vi "HexDAQ.vi"() -> ()   [LabVIEW 2016]
doc: "This is the main VI for the HexDAQ project. Contains the front panel controls steers the entire data taking, logging and display."
uses:
  input_params.ctl
  refs_front_panel.ctl
  <extravilib>/ChannelInstances/Tag-a[.](c(a[.](stamp),a[.](dbl)))/Read With Abort.vi
  <extravilib>/ChannelInstances/Tag-bool/Read With Abort.vi
  <extravilib>/ChannelInstances/Tag-t'input_params.ctl'/Write With Abort.vi
  <extravilib>/ChannelInstances/Tag-str/Write With Abort.vi
  <extravilib>/ChannelInstances/Tag-bool/Write With Abort.vi
  <extravilib>/ChannelInstances/Tag-t'data_env.ctl'/Instantiate.vi
  <extravilib>/ChannelInstances/Tag-t'input_params.ctl'/Instantiate.vi
  <extravilib>/ChannelInstances/Tag-str/Instantiate.vi
  <extravilib>/ChannelInstances/Tag-a[.](c(a[.](stamp),a[.](dbl)))/Instantiate.vi
  <extravilib>/ChannelInstances/Tag-bool/Instantiate.vi
  <extravilib>/ChannelInstances/Tag-a[.](c(a[.](stamp),a[.](dbl)))/EndpointRead.vi
  <extravilib>/ChannelInstances/Tag-bool/EndpointRead.vi
  <extravilib>/ChannelInstances/Tag-t'input_params.ctl'/Endpoint.vi
  <extravilib>/ChannelInstances/Tag-str/Endpoint.vi
  <extravilib>/ChannelInstances/Tag-bool/Endpoint.vi
  <extravilib>/ChannelInstances/Tag-bool.lvlib
  <extravilib>/ChannelInstances/Tag-a[.](c(a[.](stamp),a[.](dbl))).lvlib
  <extravilib>/ChannelInstances/Tag-str.lvlib
  user32.dll
  <extravilib>/ChannelInstances/Tag-t'input_params.ctl'.lvlib
panel:
  in  "Mask pad above (uA)":dbl=1.0
  in  "Mask pads":string
  in  "Source interlock?":bool=TRUE
  out "Missing current [%]\n(Sum cells - tot)/tot":dbl format="%#.0f"
  in  "Abort 3":bool
  in  "END DAQ 2":bool
  in  "Polarity: switch only affects contact test to be forward bias always.":enum32{"Radio Selection 1", "Radio Selection 2"}(radio)
  in  "CV Switch Delay (s)":dbl=0.3
  in  "IV Switch Delay (s)":dbl=0.3
  in  "CV voltage file":path=path "C:/Users/Administrator/Desktop/HGCAL_sensor_tests/config/voltagesCV.txt"
  in  "IV voltage file":path=path "C:/Users/Administrator/Desktop/HGCAL_sensor_tests/config/voltagesIV.txt"
  in  "Abort 2":bool
  in  "No CV corrections":bool=TRUE
  in  "Total curr/vlt \nevery x pads":i32=10
  in  "Disable Switchcard":bool
  in  "Comments (saved in data file)":string
  in  "Needle?":bool
  out "Total current":cluster{i32[], dbl[]}[](graph) caption="XY Graph"
  in  "CV voltage delay (s)":dbl=20.0
  in  "Sensor type":T1(ring)
  in  "Custom pad scan":string
  in  "Measurement type":T2(ring)=enum."Debug"
  in  "Hex pad numbers?":bool=TRUE
  in  "?":refnum<k7>(container)
  in  "Custom\nvoltages IV":string
  out "Single channel IV/CV curve":cluster{"X array":dbl[], "Y array":dbl[]}[](graph) caption="XY Graph"
  in  "Repeat":i32=1
  in  "LCR signal voltage (V)":dbl=0.501
  in  "LCR signal frequenzy (kHz)":dbl=50.0 format="%#_13g"
  in  "Sampling number":i32=3
  in  "DMM device":T3(ring)=enum."Keithley6487"
  in  "Take environmental sensor data from":T4(ring)=enum."Switch Matrix"
  out "Environmental data":cluster{timestamp[], dbl[]}[](graph)
  out "Elapsed time":dbl format="%<%H:%M:%S>t"
  out "Estimated remaining time":dbl format="%<%H:%M:%S>t"
  out "Channel values":cluster{i32[], dbl[]}[](graph) caption="XY Graph"
  out "Current channel":dbl format="%#_13g"
  out "Current source voltage (V)":dbl format="%#_13g"
  in  "Abort":bool
  in  "Output file":refnum<k7>(container) caption="Preview data file"
  in  "END DAQ":bool
  in  "START DAQ":bool
  in  "Custom\nvoltages CV":string
  in  "Data storage location:":path=path "C:/Users/Administrator/cernbox/HGCAL test results/Data"
  in  "Plot after execution?":bool=TRUE
  in  "Voltage limit (V)":dbl=1000.0
  in  "Compliance  level (uA)":dbl=500.0
  in  "VISA resource name LCR":refnum<visa-resource-name>="LCR_E4980"
  in  "VISA resource name DMM":refnum<visa-resource-name>="KEITHLEY_6487"
  in  "VISA resource name source":refnum<visa-resource-name>="Source_2410"
  in  "IV voltage delay (s)":dbl=5.0
  in  "Display/needle\nchannel":i32=144
  in  "Open after execution?":bool
  in  "Identifier (eg. wafer number)":string="Debug"
  # "HexDAQ\nThe LabVIEW program for HGCAL sensor tests\nFeedback and bug reports to andreas.alexander.maier@cern.ch"
  # "Measurement settings"
  # "Bookkeeping settings"
  # "VISA settings"
  # "Both used to determine \nthe folder and file names"
  # "Device settings"
  # "Debug settings"
  # "Timing settings"
  # "Data processing settings"
  # "Ctrl+H for full display"
  # "p on n (no sign inversion)"
  # "n on p (inversion for contact test)"
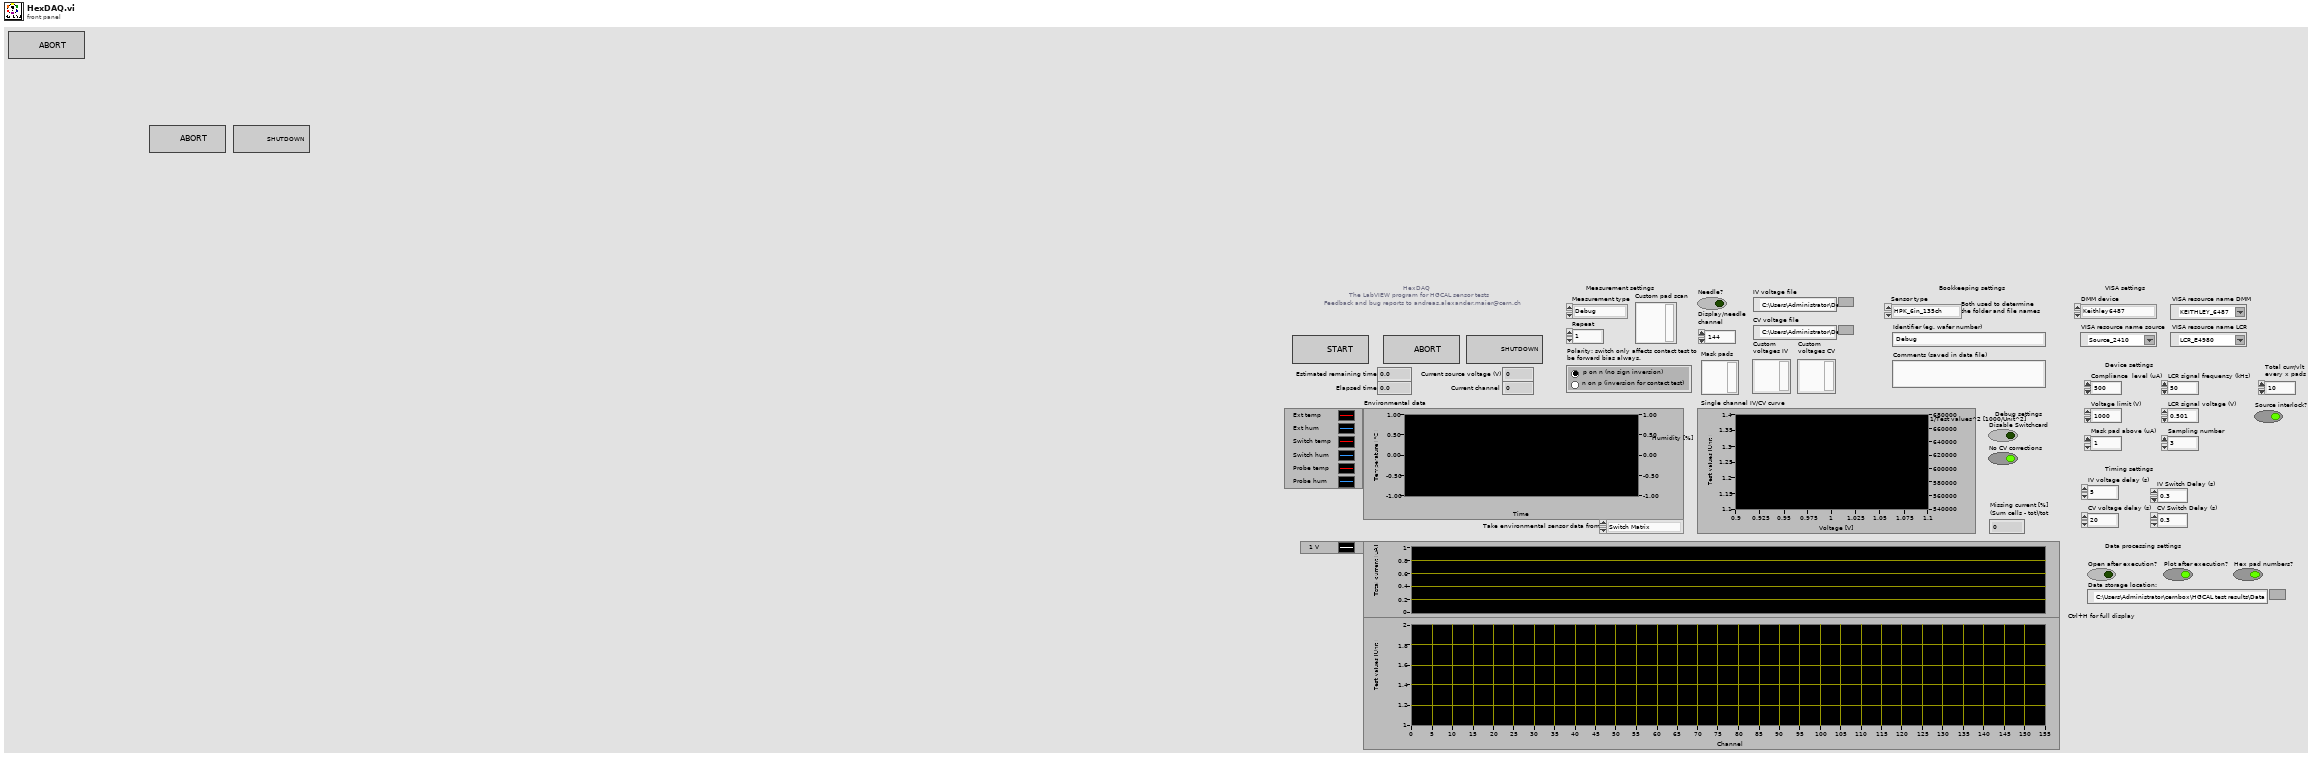
[diagram p1: front panel]
types:
  T1 = enum16{"HPK_6in_135ch", "HPK_8in_271ch", "IFX_8in_256ch", "Diode", "HPK_6in_239ch", "Full_Matrix"}
  T2 = enum16{"IV", "CV", "Debug", "Test_contact", "IV+CV"}
  T3 = enum16{"Keithley2001", "Keithley2450", "Keithley2410", "Keithley6487", "Keithley6517"}
  T4 = enum16{"Sensirion sht1x/7x", "Switch Matrix", "Probecard"}
  T5 = typedef "refs_front_panel.ctl" = cluster{"Current voltage (V)":refnum<vi>, "Elapsed time":refnum<vi>, "Current channel":refnum<vi>, "Abort":refnum<vi>, "Estimated remaining time":refnum<vi>, "Channel values XYGraph":refnum<vi>, "Single channel XYGraph":refnum<vi>, "Total current XYGraph":refnum<vi>, "Missing\ncurrent [%]":refnum<vi>}
  T6 = typedef "input_params.ctl" = cluster{"Measurement type":enum16{"IV", "CV", "Debug", "Test_contact"}, "Sensor type":enum16{"HPK_6in_135ch", "HPK_8in_271ch", "IFX_8in_256ch", "Diode", "HPK_6in_239ch", "Full_Matrix", ""}, "Identifier":string, "Open after execution?":bool, "Plot after execution?":bool, "Display channel":i32, "Voltage Delay (s)":dbl, "Switch Delay (s)":dbl, "VISA resource name source":refnum<visa-resource-name>, "VISA resource name DMM":refnum<visa-resource-name>, "VISA resource name LCR":refnum<visa-resource-name>, "Compliance  Level (A)":dbl, "Voltage Limit (V)":dbl, "Data storage location":string, "Scan voltages":string, "Use source as DMM?":bool, "LCR signal frequenzy (Hz)":dbl, "DMM device":enum16{"Keithley2001", "Keithley2450", "Keithley2410", "Keithley6487", "Keithley6517"}, "Sampling number":i32, "Use env. sensors on":enum16{"Sensirion sht1x/7x", "Switch Matrix", "Probecard"}, "Switchboard Handle":u32, "Use Switchboard":bool, "LCR signal voltage (V)":dbl, "Repeat":i32, "Scan voltages IV":string, "Scan voltages CV":string, "Hex pad numbers?":bool, "Set measurement type":enum16{"IV", "CV", "Debug", "Test_contact", "IV+CV"}, "Custom pad scan":string, "IV voltage Delay (s)":dbl, "CV voltage Delay (s)":dbl, "Needle measurement?":bool, "Comments":string, "LCR signal frequenzy (kHz)":dbl, "Compliance  Level (uA)":dbl, "Open Correction Array":dbl[][], "Current set voltage":dbl, "Last set voltage":dbl, "Current channel":i32, "Last OpenCorrection index":i32, "Total curr/vltg every x steps":i32, "Current channel iteration":i32, "No CV corrections":bool, "Mapfile":string, "Corrfile":string, "IV voltage file":path, "CV voltage file":path, "IV Switch Delay (s)":dbl, "CV Switch Delay (s)":dbl, "Invert polarity":bool, "Set debug dirs":bool, "Is n on p":bool, "Source interlock?":bool, "Voltage file used?":bool, "Pad mask":string, "Mask pad above (uA)":dbl}
  T7 = typedef "Tag-t'input_params.ctl'.lvlib/))Channel.ctl" = refnum<queue>
  T8 = typedef "Tag-str.lvlib/))Channel.ctl" = refnum<queue>
  T9 = typedef "data_dynamic.ctl" = cluster{"Output file":path, "Y-label text":string, "Current set voltage":dbl, "Set voltage column":dbl[], "Pad number column":dbl[], "Data  column":dbl[], "Number of voltages":i32, "Compliance current (A)":dbl, "Geofile":string, "Peak voltage":dbl, "Hex PDF file":string, "Voltage array":dbl[], "Total current column":dbl[], "Timestamp column":dbl[], "Data name":string, "Data unit":string, "2nd data column":dbl[], "2nd data name":string, "2nd data unit":string, "3rd data column":dbl[], "4th data column":dbl[], "3rd data name":string, "3rd data unit":string, "4th data name":string, "4th data unit":string, "Actual voltage column":dbl[], "2nd Y-label text":string, "Single channel plot":path, "Temperature column":dbl[], "Humidity column":dbl[], "Channel switch array":i32[], "1st single plot name":string, "2nd single plot name":string, "All channels plot":path, "HexPlot command":string, "Custom channel array":i32[], "Data  error column":dbl[], "2nd data  error column":dbl[], "3rd data error column":dbl[], "4th data  error column":dbl[], "Total current plot":path, "5th data column":dbl[], "5th data  error column":dbl[], "6th data column":dbl[], "6th data  error column":dbl[], "5th data name":string, "5th data unit":string, "6th data name":string, "6th data unit":string, "HexPlot matrix command":string}
  T10 = typedef "Tag-bool.lvlib/))Channel.ctl" = refnum<queue>
  T11 = typedef "Tag-a[.](c(a[.](stamp),a[.](dbl))).lvlib/))Channel.ctl" = refnum<queue>
  T12 = typedef "Tag-t'data_env.ctl'.lvlib/))Channel.ctl" = refnum<queue>
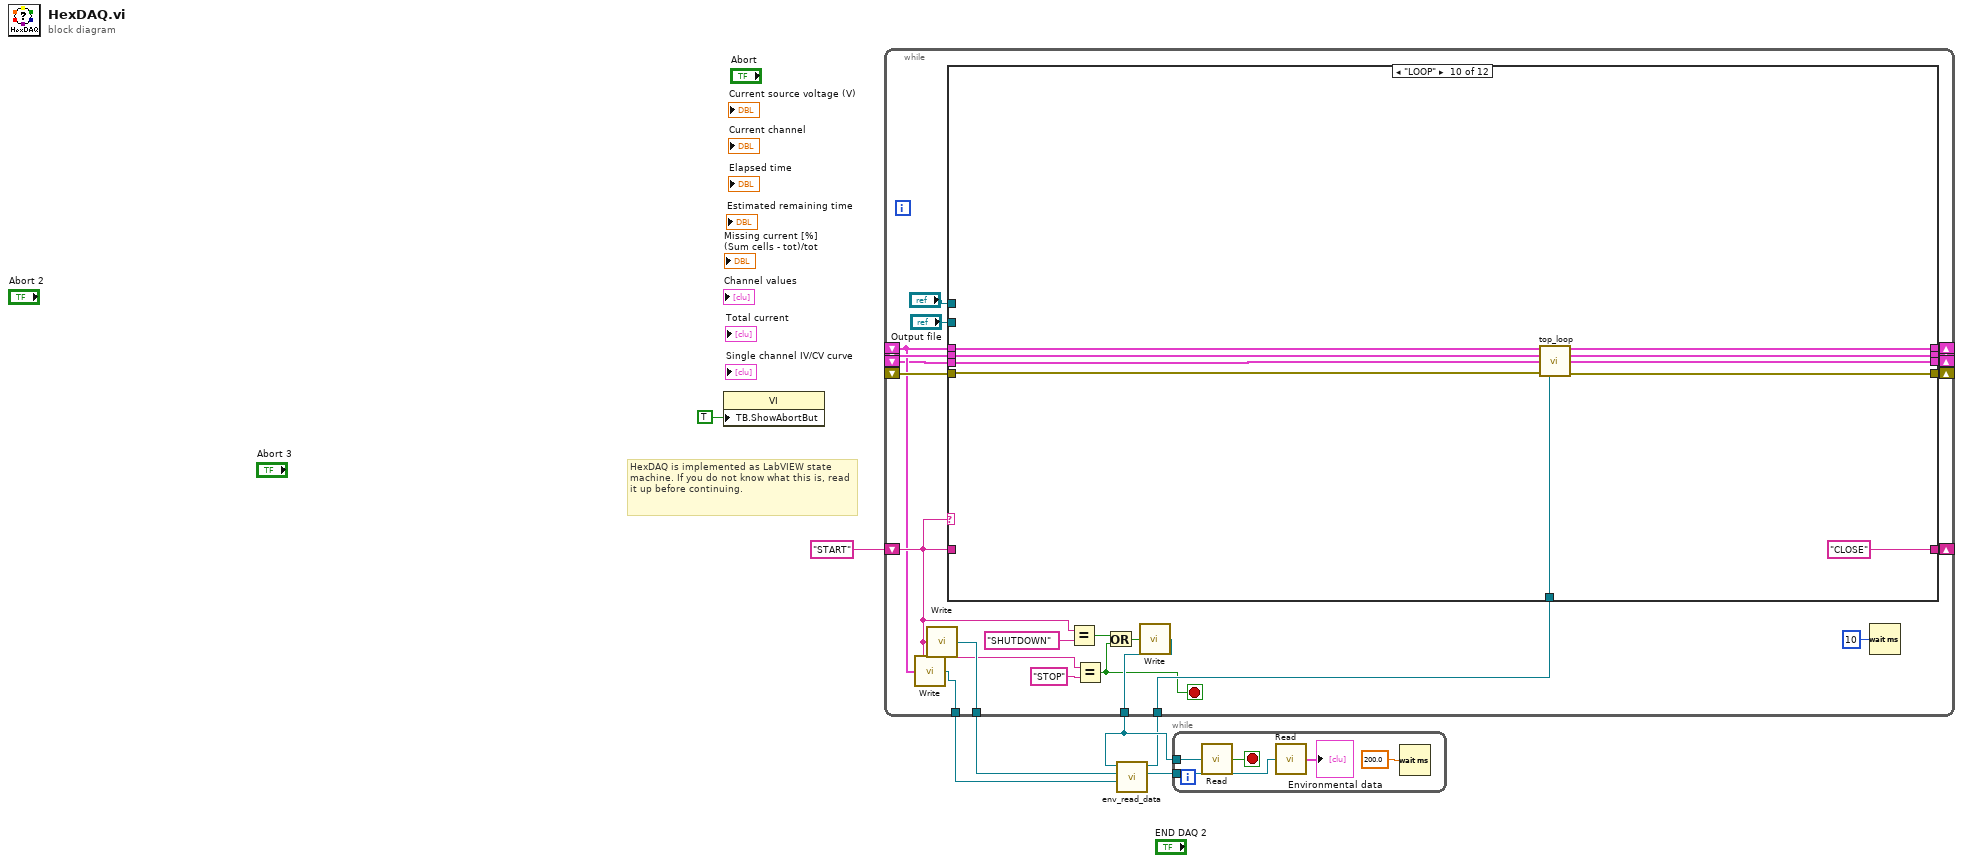
[diagram p0: block diagram]
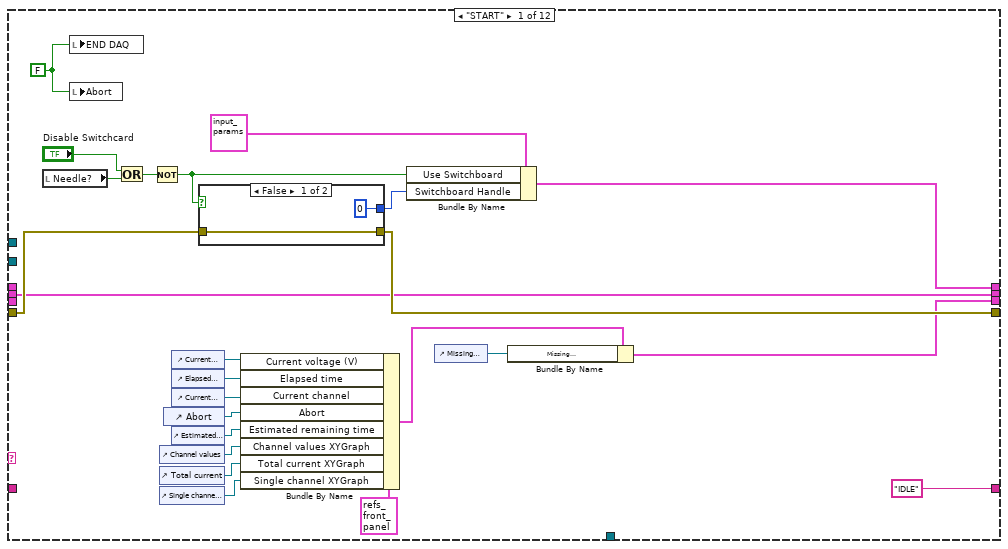
[diagram p2: hidden frame]
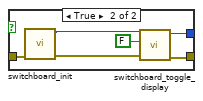
[diagram p3: hidden frame]
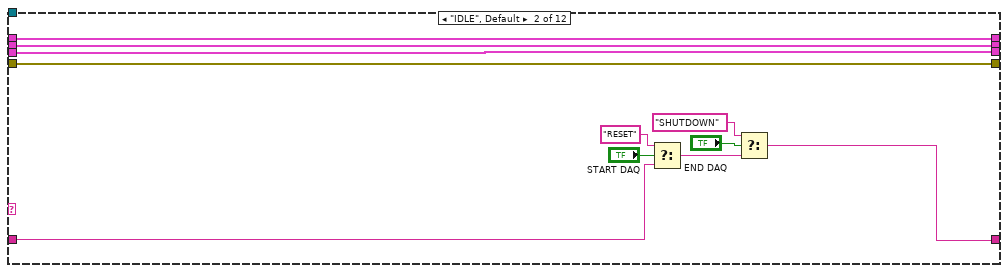
[diagram p4: hidden frame]
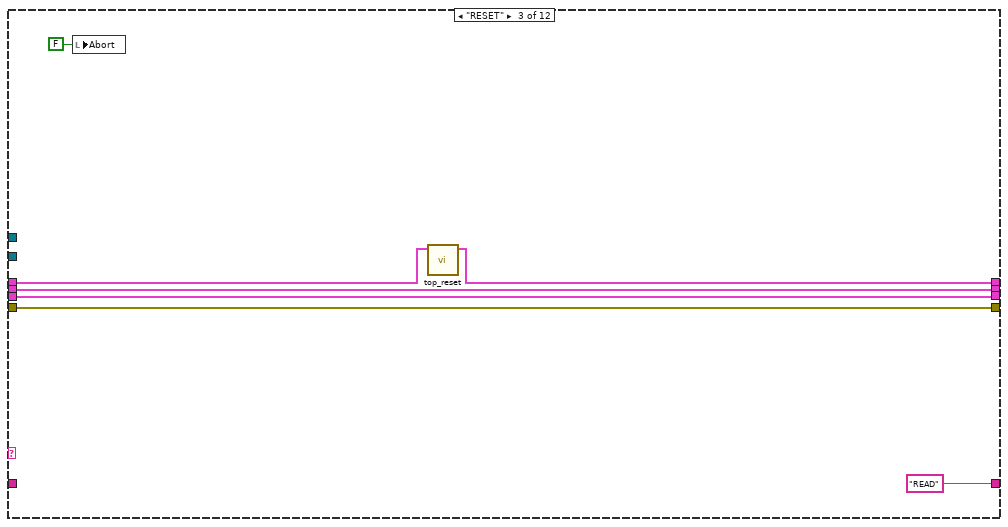
[diagram p5: hidden frame]
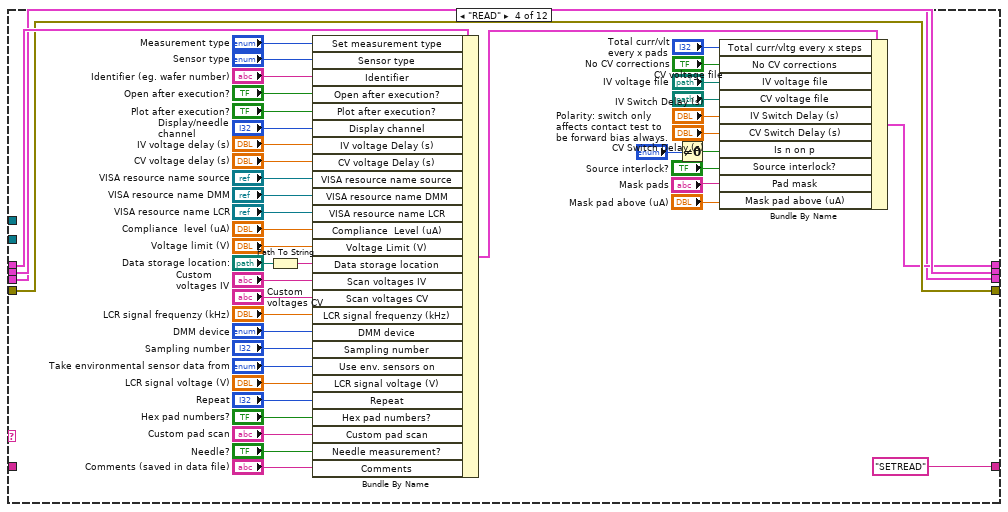
[diagram p6: hidden frame]
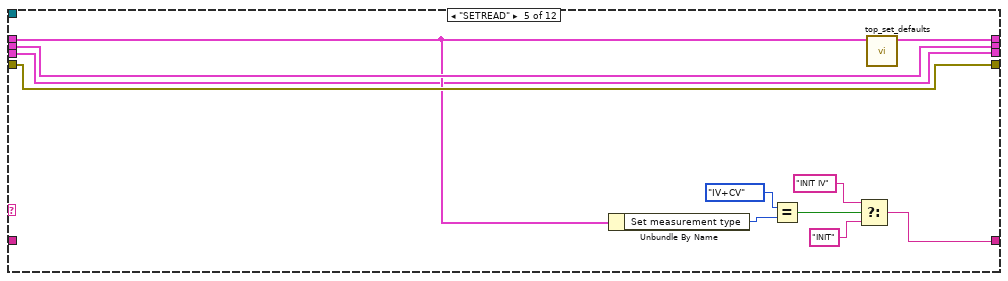
[diagram p7: hidden frame]
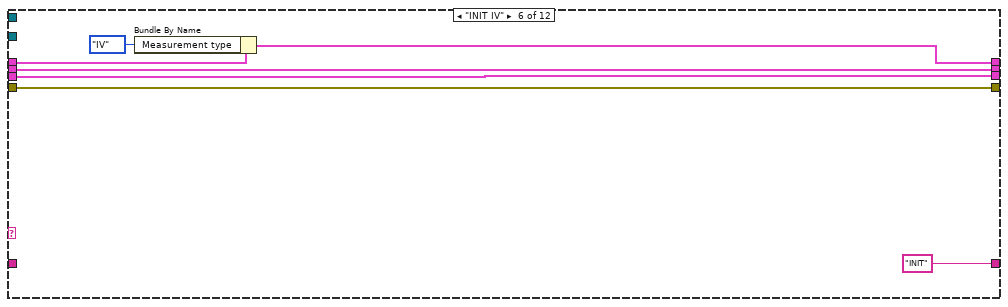
[diagram p8: hidden frame]
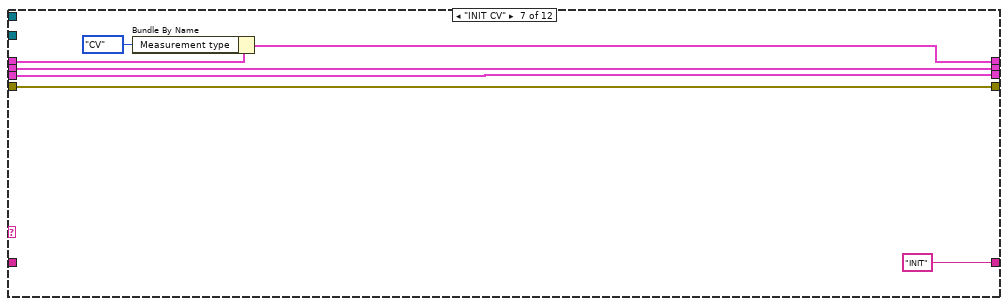
[diagram p9: hidden frame]
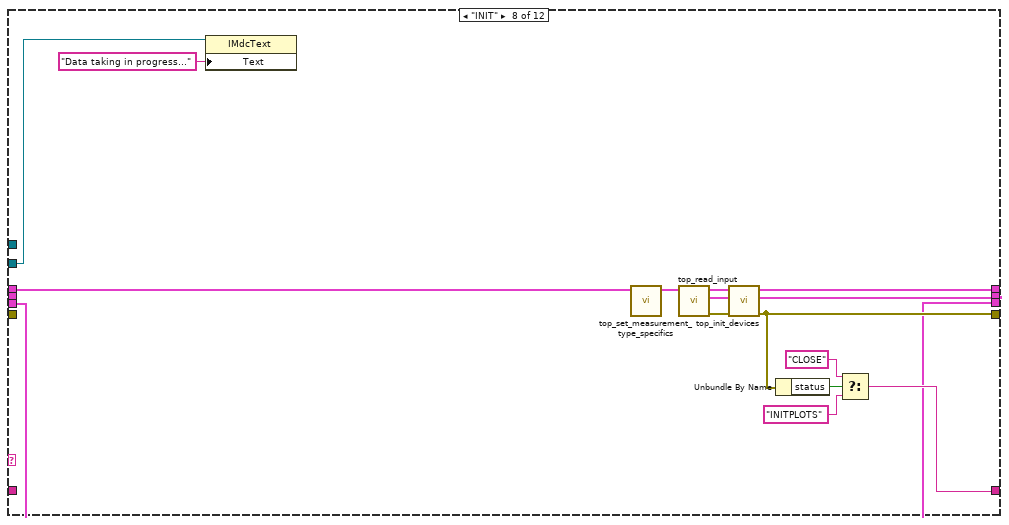
[diagram p10: hidden frame]
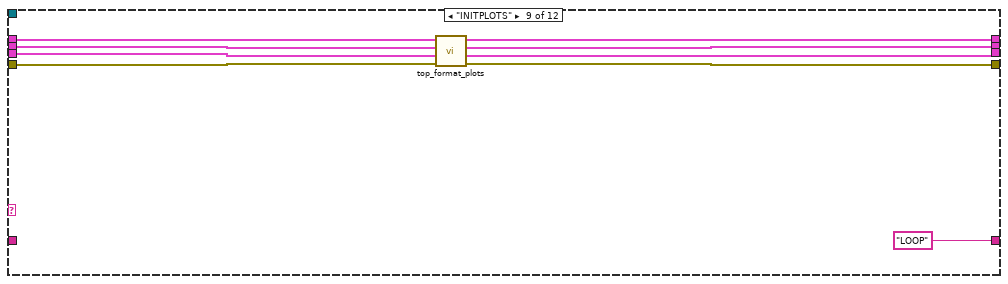
[diagram p11: hidden frame]
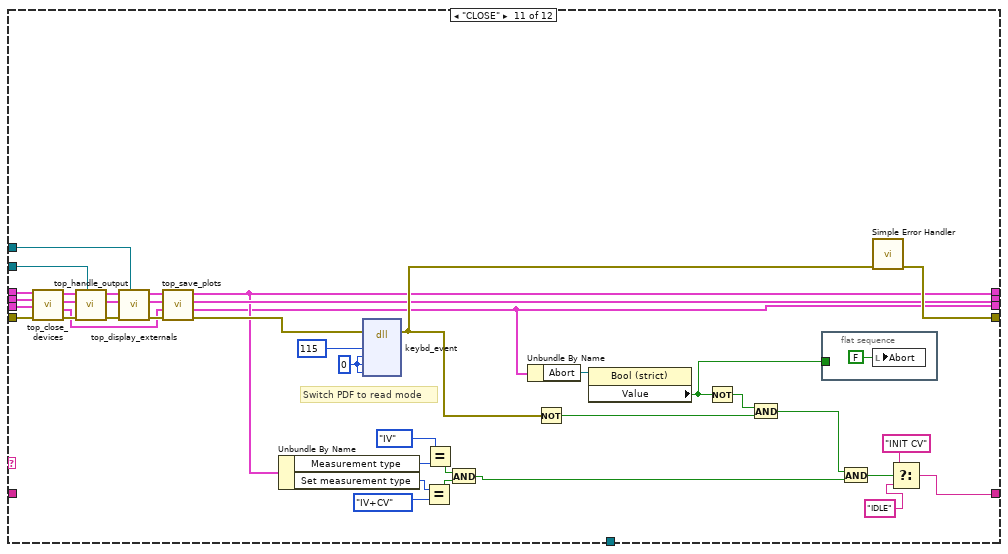
[diagram p12: hidden frame]
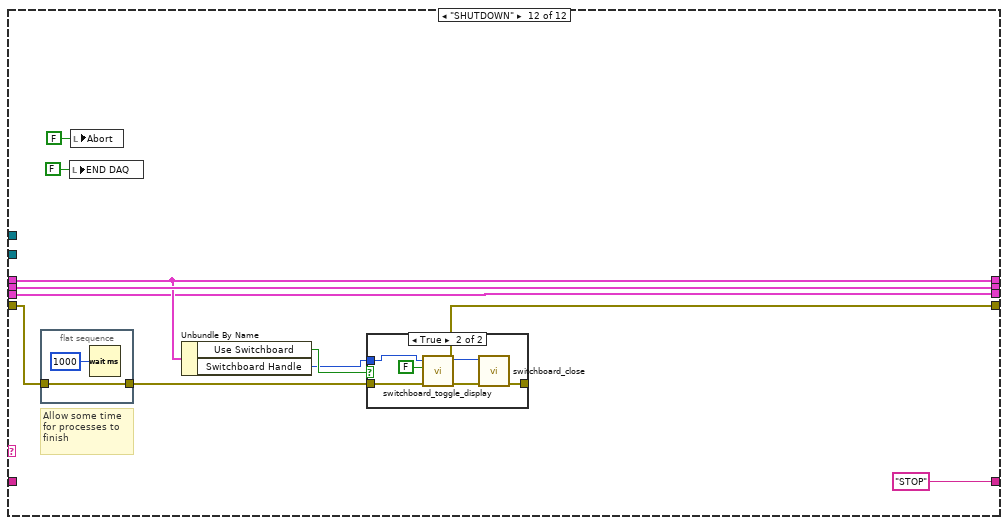
[diagram p13: hidden frame]
diagram:
  # "HexDAQ is implemented as LabVIEW state machine. If you do not know what this is, read it up before continuing."
  n1 = property class="VI"("TB.ShowAbortBut"=TRUE ("Tool Bar:Show Abort Button")) -> ()  [unwired: 2 in, 2 out]
  n2 = while {
    shift-right: [w29] -> _
    shift-left: "START" -> [w16]
    shift-right: [w24] -> _
    shift-left: _ -> [w22]
    shift-right: [w26] -> _
    shift-left: _ -> [w23]
    shift-right: [w25] -> _
    shift-left: _ -> [w12]
    tunnel: [w21] -> w5
    tunnel: w1 -> [w19]
    tunnel: [w18] -> w3
    tunnel: [w8] -> w2
    shift-right: [w10] -> _
    shift-left: _ -> [w9]
    stop <- w13 stop-if-true
    n3 = call <extravilib>:"Write.vi"("element"=w12) -> ("channel"=w8:T7)  [unwired: 1 out]
    n4 = call <extravilib>:"Write.vi"("element"=w16) -> ("channel"=w18:T8)  [unwired: 1 out]
    n5 = case shown="\"LOOP\"" w16 {
      tunnel: w16 -> [_ w72 _ _ _ _ _ _ _ _ _ _]
      tunnel: ["IDLE" ("t") w69 "READ" ("t") "SETREAD" ("t") w130 "INIT" ("t") "INIT" ("t") w153 "LOOP" ("t") "CLOSE" ("t") w202 "STOP" ("t")] -> w29
      tunnel: [w47 w65 w74 w92 w127 w139 w146 w161 w169 w182 w192 w227] -> w25
      tunnel: [w51 w64 w78 w102 w134 w142 w149 w157 w165 w180 w215 w231] -> w24
      tunnel: [w48 w63 w75 w103 w135 w141 w148 w160 w168 w181 w194 w234] -> w26
      tunnel: w12 -> [_ w65 w73 w104 w126 w140 w147 w151 w172 w177 w217 w227]
      tunnel: w23 -> [w48 w63 w75 w103 w135 w141 w148 _ w173 w178 w212 w234]
      tunnel: w22 -> [w52 w64 w78 w102 w134 w142 w149 _ w166 w179 w216 w229]
      tunnel: "Output file" -> [_ _ _ _ _ _ _ w158 _ _ w214 _]
      tunnel: "?" -> [_ _ _ _ _ _ _ _ _ _ w213 _]
      tunnel: w19 -> [_ _ _ _ _ _ _ _ _ w176 _ _]
      tunnel: [w32 w62 w77 w89 w125 w136 w143 w152 w167 w175 w191 w226] -> w10
      tunnel: w9 -> [_ w62 w77 w89 w125 w136 w143 w152 w170 w174 w185 w226]
      frame "START" {
        w33 = FALSE ("Abort")
        n6 = local read "Needle?"() -> (w44:bool)
        n7 = local write "END DAQ"(w33) -> ()
        n8 = local write "Abort"(w33) -> ()
        n9 = Or(x="Disable Switchcard", y=w44) -> (x .or. y?=w43:bool)
        n10 = Not(x=w43) -> (.not. x?=w46:bool)
        n11 = control-ref of="Channel values"() -> (w36:refnum<vi>)
        n12 = control-ref of="Total current"() -> (w35:refnum<vi>)
        n13 = control-ref of="Single channel IV/CV curve"() -> (w34:refnum<vi>)
        n14 = control-ref of="Abort"() -> (w38:refnum<vi>)
        n15 = control-ref of="Current source voltage (V)"() -> (w40:refnum<vi>)
        n16 = control-ref of="Elapsed time"() -> (w41:refnum<vi>)
        n17 = control-ref of="Current channel"() -> (w39:refnum<vi>)
        n18 = control-ref of="Estimated remaining time"() -> (w37:refnum<vi>)
        n19 = case shown="False" w46 {
          tunnel: w52 -> [w55 w61]
          tunnel: [w55 w60] -> w51
          tunnel: [u32 0 ("Handle") w58] -> w50
          frame False {
          }
          frame True {
            n20 = call <instrlib>:"switchboard_init.vi"("error in"=w61) -> ("error out"=w57:errorcluster, "Handle"=w56:u32)  [unwired: 9 in]
            n21 = call <instrlib>:"switchboard_toggle_display.vi"("error in"=w57, "On/Off"=FALSE, "Handle"=w56) -> ("error out"=w60:errorcluster, "Handle out"=w58:u32)  [unwired: 7 in]
          }
        }
        n22 = Bundle By Name(cluster=T5 {"Current voltage (V)"=refnum, "Elapsed time"=refnum, "Current channel"=refnum, "Abort"=refnum, "Estimated remaining time"=refnum, "Channel values XYGraph"=refnum, "Single channel XYGraph"=refnum, "Total current XYGraph"=refnum, "Missing\ncurrent [%]"=refnum} ("Cluster"), "Current voltage (V)"=w40, "Elapsed time"=w41, "Current channel"=w39, "Abort"=w38, "Estimated remaining time"=w37, "Channel values XYGraph"=w36, "Total current XYGraph"=w35, "Single channel XYGraph"=w34) -> (w31:T5)
        n23 = Bundle By Name(cluster=T6 {"Measurement type"=enum."Debug", "Sensor type"=enum."HPK_6in_135ch", "Identifier"="test.txt", "Open after execution?"=FALSE, "Plot after execution?"=FALSE, "Display channel"=0, "Voltage Delay (s)"=0.5, "Switch Delay (s)"=0.01, "VISA resource name source"="", "VISA resource name DMM"="", "VISA resource name LCR"="", "Compliance  Level (A)"=10.0, "Voltage Limit (V)"=1000.0, "Data storage location"="", "Scan voltages"="", "Use source as DMM?"=FALSE, "LCR signal frequenzy (Hz)"=10.0, "DMM device"=enum."Keithley2001", "Sampling number"=1, "Use env. sensors on"=enum."Sensirion sht1x/7x", "Switchboard Handle"=0, "Use Switchboard"=FALSE, "LCR signal voltage (V)"=10000.0, "Repeat"=1, "Scan voltages IV"="", "Scan voltages CV"="", "Hex pad numbers?"=FALSE, "Set measurement type"=enum."Debug", "Custom pad scan"="", "IV voltage Delay (s)"=0.5, "CV voltage Delay (s)"=0.5, "Needle measurement?"=FALSE, "Comments"="test.txt", "LCR signal frequenzy (kHz)"=10.0, "Compliance  Level (uA)"=10.0, "Open Correction Array"=array2304x3[6912 elements], "Current set voltage"=0.0, "Last set voltage"=0.0, "Current channel"=0, "Last OpenCorrection index"=-1, "Total curr/vltg every x steps"=10, "Current channel iteration"=0, "No CV corrections"=FALSE, "Mapfile"="", "Corrfile"="", "IV voltage file"=path "", "CV voltage file"=path "", "IV Switch Delay (s)"=0.01, "CV Switch Delay (s)"=0.01, "Invert polarity"=FALSE, "Set debug dirs"=FALSE, "Is n on p"=FALSE, "Source interlock?"=TRUE, "Voltage file used?"=FALSE, "Pad mask"="", "Mask pad above (uA)"=1.0} ("Input parameters"), "Use Switchboard"=w46, "Switchboard Handle"=w50) -> (w47:T6)
        n24 = control-ref of="Missing current [%]\n(Sum cells - tot)/tot"() -> (w30:refnum<vi>)
        n25 = Bundle By Name(cluster=w31, "Missing\ncurrent [%]"=w30) -> (w32:T5)
      }
      frame "IDLE", Default {
        n26 = Select(t="RESET", s="START DAQ", f=w72) -> (s? t:f=w70:string)
        n27 = Select(t="SHUTDOWN", s="END DAQ", f=w70) -> (s? t:f=w69:string)
      }
      frame "RESET" {
        n28 = local write "Abort"(FALSE ("Abort")) -> ()
        n29 = call "top_reset.vi"("Input parameters"=w73) -> ("New input parameters"=w74:T6)  [unwired: 10 in]
      }
      frame "READ" {
        n30 = Path To String(path="Data storage location:") -> (string=w107:string)
        n31 = Bundle By Name(cluster=w104, "Set measurement type"="Measurement type", "Sensor type"="Sensor type", "Identifier"="Identifier (eg. wafer number)", "Open after execution?"="Open after execution?", "Plot after execution?"="Plot after execution?", "Display channel"="Display/needle\nchannel", "IV voltage Delay (s)"="IV voltage delay (s)", "CV voltage Delay (s)"="CV voltage delay (s)", "VISA resource name source"="VISA resource name source", "VISA resource name DMM"="VISA resource name DMM", "VISA resource name LCR"="VISA resource name LCR", "Compliance  Level (uA)"="Compliance  level (uA)", "Voltage Limit (V)"="Voltage limit (V)", "Data storage location"=w107, "Scan voltages IV"="Custom\nvoltages IV", "Scan voltages CV"="Custom\nvoltages CV", "LCR signal frequenzy (kHz)"="LCR signal frequenzy (kHz)", "DMM device"="DMM device", "Sampling number"="Sampling number", "Use env. sensors on"="Take environmental sensor data from", "LCR signal voltage (V)"="LCR signal voltage (V)", "Repeat"="Repeat", "Hex pad numbers?"="Hex pad numbers?", "Custom pad scan"="Custom pad scan", "Needle measurement?"="Needle?", "Comments"="Comments (saved in data file)") -> (w93:T6)
        n32 = Not Equal To 0?(x="Polarity: switch only affects contact test to be forward bias always.") -> (x != 0?=w84:bool)
        n33 = Bundle By Name(cluster=w93, "Total curr/vltg every x steps"="Total curr/vlt \nevery x pads", "No CV corrections"="No CV corrections", "IV voltage file"="IV voltage file", "CV voltage file"="CV voltage file", "IV Switch Delay (s)"="IV Switch Delay (s)", "CV Switch Delay (s)"="CV Switch Delay (s)", "Is n on p"=w84, "Source interlock?"="Source interlock?", "Pad mask"="Mask pads", "Mask pad above (uA)"="Mask pad above (uA)") -> (w92:T6)
      }
      frame "SETREAD" {
        n34 = Unbundle By Name(w126) -> ("Set measurement type"=w128:T2)
        n35 = Equal?(x=T2."IV+CV" ("Measurement type"), y=w128) -> (x = y?=w129:bool)
        n36 = Select(t="INIT IV", s=w129, f="INIT" ("t")) -> (s? t:f=w130:string)
        n37 = call "top_set_defaults.vi"("Input parameters"=w126) -> ("Input parameters out"=w127:T6)  [unwired: 10 in]
      }
      frame "INIT IV" {
        n38 = Bundle By Name(cluster=w140, "Measurement type"=enum16{"IV", "CV", "Debug", "Test_contact"}."IV") -> (w139:T6)
      }
      frame "INIT CV" {
        n39 = Bundle By Name(cluster=w147, "Measurement type"=enum16{"IV", "CV", "Debug", "Test_contact"}."CV") -> (w146:T6)
      }
      frame "INIT" {
        n40 = property class="IMdcText"(reference=w158, "Text"="Data taking in progress...") -> ()  [unwired: 1 in, 2 out]
        n41 = call "top_set_measurement_type_specifics.vi"("Input parameters"=w151) -> ("Input parameters out"=w150:T6)  [unwired: 10 in]
        n42 = call "top_read_input.vi"("Input parameters"=w150) -> ("error out"=w163:errorcluster, "Dynamic data"=w162:T9, "Input parameters"=w164:T6)  [unwired: 8 in]
        n43 = call "top_init_devices.vi"("error in (no error)"=w163, "Dynamic data"=w162, "Input parameters"=w164) -> ("error out"=w157:errorcluster, "Dynamic data"=w160:T9, "Input parameters"=w161:T6)  [unwired: 6 in]
        n44 = Unbundle By Name(w157) -> ("status"=w156:bool)
        n45 = Select(t="CLOSE", s=w156, f="INITPLOTS" ("t")) -> (s? t:f=w153:string)
      }
      frame "INITPLOTS" {
        n46 = call "top_format_plots.vi"("error in"=w166, "Front panel refs"=w170, "Dynamic data"=w173, "Input parameters"=w172) -> ("error out"=w165:errorcluster, "Front panel refs out"=w167:T5, "Dynamic data out"=w168:T9, "Input parameters out"=w169:T6)  [unwired: 4 in]
      }
      frame "LOOP" {
        n47 = call "top_loop.vi"("Input parameters"=w177, "Dynamic data"=w178, "Front_panel_refs"=w174, "error in (no error)"=w179, "Environmental data"=w176) -> ("Input parameters out"=w182:T6, "Dynamic data out"=w181:T9, "Front_panel_refs out"=w175:T5, "error out"=w180:errorcluster)  [unwired: 7 in]
      }
      frame "CLOSE" {
        w199 = u8 0 ("bScan")
        # "Switch PDF to read mode"
        n48 = call "top_close_devices.vi"("error in (no error)"=w216, "Front_panel_refs"=w185, "Dynamic data"=w212, "Input parameters"=w217) -> ("error out"=w223:errorcluster, "Front_panel_refs out"=w184:T5, "Dynamic data"=w221:T9, "Input parameters"=w222:T6)  [unwired: 4 in]
        n49 = call "top_handle_output.vi"("Output file text box"=w214, "error in (no error)"=w223, "Dynamic data"=w221, "Input parameters"=w222) -> ("error out"=w220:errorcluster, "Dynamic data"=w219:T9, "Input parameters"=w218:T6)  [unwired: 5 in]
        n50 = call "top_display_externals.vi"("AcroPDF"=w213, "error in (no error)"=w220, "Dynamic data"=w219, "Input parameters"=w218) -> ("error out"=w211:errorcluster, "Dynamic data"=w195:T9, "Input parameters"=w193:T6)  [unwired: 5 in]
        n51 = call "top_save_plots.vi"("error in"=w211, "Front_panel_refs"=w184, "Dynamic data"=w195, "Input parameters"=w193) -> ("error out"=w197:errorcluster, "Front_panel_refs out"=w191:T5, "Dynamic data out"=w194:T9, "Input parameters out"=w192:T6)  [unwired: 4 in]
        n52 = Unbundle By Name(w192) -> ("Measurement type"=w210:enum16{"IV", "CV", "Debug", "Test_contact"}, "Set measurement type"=w208:T2)
        n53 = dll-call lib="user32.dll" fn="keybd_event"(error in=w197, "bVk"=u8 115 ("Virtual Key"), "bScan"=w199, "dwFlags"=w199, "dwExtraInfo"=w199) -> (error out=w196:errorcluster)  [unwired: 7 in, 1 out]
        n54 = Equal?(x=w208, y=T2."IV+CV") -> (x = y?=w205:bool)
        n55 = Equal?(x=enum16{"IV", "CV", "Debug", "Test_contact"}."IV", y=w210) -> (x = y?=w206:bool)
        n56 = And(x=w206, y=w205) -> (x .and. y?=w187:bool)
        n57 = Unbundle By Name(w191) -> ("Abort"=w190:refnum<vi>)
        n58 = Not(x=w196) -> (.not. x?=w188:bool)
        n59 = property class="Bool (strict)"(reference=w190) -> ("Value"=w201:bool)  [unwired: 1 in, 2 out]
        n60 = Not(x=w201) -> (.not. x?=w189:bool)
        n61 = And(x=w189, y=w188) -> (x .and. y?=w186:bool)
        n62 = flat-sequence {
          tunnel: w201 -> [_]
          frame #0 {
            n63 = local write "Abort"(FALSE ("Abort")) -> ()
          }
        }
        n64 = And(x=w186, y=w187) -> (x .and. y?=w200:bool)
        n65 = call <vilib>:"Simple Error Handler.vi"("error in (no error)"=w196) -> ("error out"=w215:errorcluster)  [unwired: 4 in, 4 out]
        n66 = Select(t="INIT CV", s=w200, f="IDLE" ("t")) -> (s? t:f=w202:string)
      }
      frame "SHUTDOWN" {
        # "Allow some time\nfor processes to\nfinish"
        n67 = flat-sequence {
          tunnel: w229 -> [w236]
          tunnel: [w236] -> w228
          frame #0 {
            n68 = Wait (ms)(milliseconds to wait=u32 1000) -> ()  [unwired: 1 out]
          }
        }
        n69 = local write "END DAQ"(FALSE ("END DAQ")) -> ()
        n70 = local write "Abort"(FALSE ("Abort")) -> ()
        n71 = Unbundle By Name(w227) -> ("Use Switchboard"=w233:bool, "Switchboard Handle"=w232:u32)
        n72 = case shown="True" w233 {
          tunnel: w228 -> [w238 w242]
          tunnel: [w238 w244] -> w231
          tunnel: w232 -> [_ w241]
          frame False {
          }
          frame True {
            n73 = call <instrlib>:"switchboard_toggle_display.vi"("error in"=w242, "On/Off"=FALSE, "Handle"=w241) -> ("error out"=w239:errorcluster, "Handle out"=w240:u32)  [unwired: 7 in]
            n74 = call <instrlib>:"switchboard_close.vi"("error in"=w239, "Handle"=w240) -> ("error out"=w244:errorcluster)  [unwired: 8 in, 1 out]
          }
        }
      }
    }
    n75 = Equal?(x=w16, y="SHUTDOWN") -> (x = y?=w15:bool)
    n76 = Equal?(x=w16, y="STOP") -> (x = y?=w13:bool)
    n77 = Or(x=w15, y=w13) -> (x .or. y?=w14:bool)
    n78 = call <extravilib>:"Write.vi"("element"=w14) -> ("channel"=w21:T10)  [unwired: 1 out]
    n79 = Wait (ms)(milliseconds to wait=u32 10) -> ()  [unwired: 1 out]
  }
  n80 = call "env_read_data.vi"("Input parameters"=w2, "State"=w3, "Stop signal"=w5) -> ("Plot data out"=w4:T11, "channel"=w1:T12)  [unwired: 6 in, 1 out]
  n81 = while {
    tunnel: w5 -> [w247]
    tunnel: w4 -> [w245]
    stop <- w246 stop-if-true
    n82 = call <extravilib>:"Read.vi"("channel"=w247) -> ("element"=w246:bool)  [unwired: 1 in, 1 out]
    n83 = call <extravilib>:"Read.vi"("channel"=w245) -> ("element"=→"Environmental data":cluster{timestamp[], dbl[]}[])  [unwired: 1 in, 1 out]
    n84 = Wait (ms)(milliseconds to wait=sgl 200.0 ("Sample period (s)")) -> ()  [unwired: 1 out]
  }
